vi "IMU Get Angular Rate.vi"(8 "error in (no error)":errorcluster) -> (0 "error out":errorcluster, 2 "timestamp":i64, 3 "rates":cluster{"x":dbl, "y":dbl, "z":dbl}(graph))   [LabVIEW 2026, in "MrcLib.lvlib"]
doc: "Returns the instantaneous rate of turn for the built-in sensor."
uses:
  MrcLib.lvlib
  Types/MRC Gyro Rates Values.ctl
panel:
  out "rates":T1
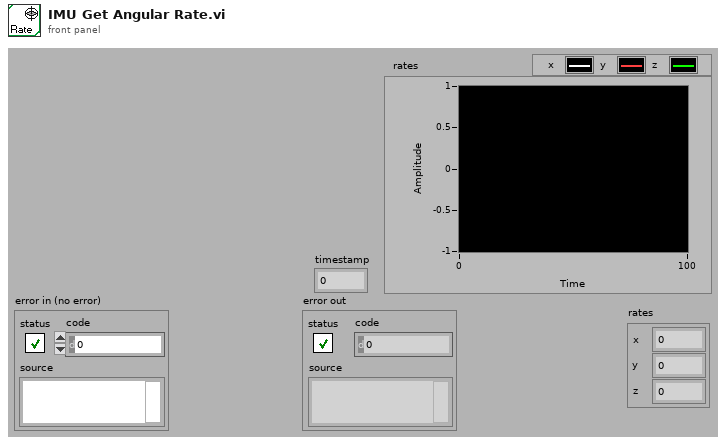
[diagram p1: front panel]
types:
  T1 = typedef "MrcLib.lvlib/MRC Gyro Rates Values.ctl" = cluster{"x":dbl, "y":dbl, "z":dbl}
  T2 = typedef "MrcLib.lvlib/MRC Gyro Rates.ctl" = cluster{"timestamp":i64, "x":dbl, "y":dbl, "z":dbl}
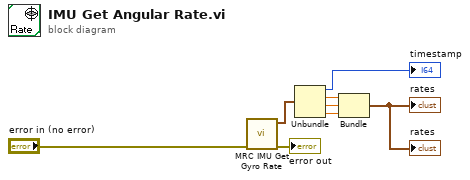
[diagram p0: block diagram]
diagram:
  n1 = call "MRC IMU Get Gyro Rate.vi"("error in (no error)"="error in (no error)") -> ("error out"=→"error out":errorcluster, "gyro rates out"=w6:T2)  [unwired: 9 in]
  n2 = Unbundle(w6) -> ("timestamp"=→"timestamp":i64, "x"=w5:dbl, "y"=w4:dbl, "z"=w3:dbl)
  n3 = Bundle("x"=w5, "y"=w4, "z"=w3) -> (→"rates" →"rates":cluster{"x":dbl, "y":dbl, "z":dbl})  [unwired: 1 in]
